vi "SD Card_Read LED  File.vi"() -> ()   [LabVIEW 2015]
doc: "TheSD Card - Read Data - Arduino Target example demonstrates how to read data previously saved in a SD Card Shield and send the data up to a Host VI via serial communication. This VI will run embedded in the Arduino target.\nTo save data in the SD Card Shield, refer to the SD Card - Log Data.vi shipping example.\n\n<b>Chip Select Pin</b>: Refer to your specific SD Card Shield documentation for its Chip Select (CS) pin number."
uses:
  <vilib>/Aledyne-TSXperts/Arduino Compatible Compiler for LabVIEW/Code Generator/Arduino APIs/Serial/Serial Settings.ctl
  <vilib>/Aledyne-TSXperts/Arduino Compatible Compiler for LabVIEW/Code Generator/Arduino APIs/SD Card/File Mode.ctl
  <vilib>/Aledyne-TSXperts/Arduino Compatible Compiler for LabVIEW/Arduino Compatible Compiler for LabVIEW.lvlib
panel:
  in  "Chip Select Pin":u8=4
  # "Overview: Demonstrates how to read data previously saved in a SD Card Shield and send the data up to a Host VI via serial communication. This VI will run embedded in the Arduino target.\n\nInstructions:\n1. Make sure the shipping example SD Card - Log Data.vi has been executed first by following its instructions. \n2. Connect the Arduino target to the PC via USB cable\n3. Enter the appropriate Chip Select as indicated in your SD Card Shield\ndocumentation\n4. Open the SD Card - Read Data - Host PC.vi and follow its instuctions\n5. Important:  This VI will be compiled and downloaded via a API call in the SD Card - Read Data - Host PC.vi. There is no need to run this VI through depressing its run button"
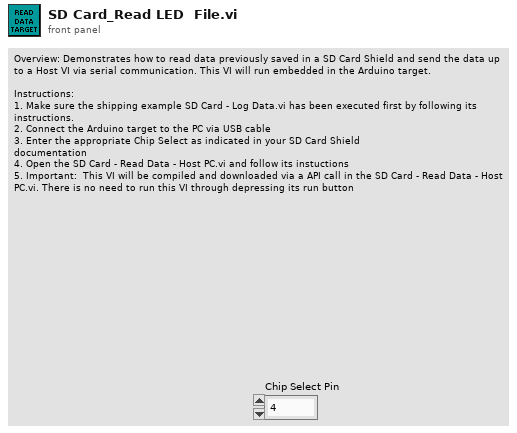
[diagram p1: front panel]
types:
  T1 = typedef "Arduino Compatible Compiler for LabVIEW.lvlib/File Mode.ctl" = enum16{"Read", "Write_Read"}
  T2 = typedef "Arduino Compatible Compiler for LabVIEW.lvlib/Serial Settings.ctl" = u16
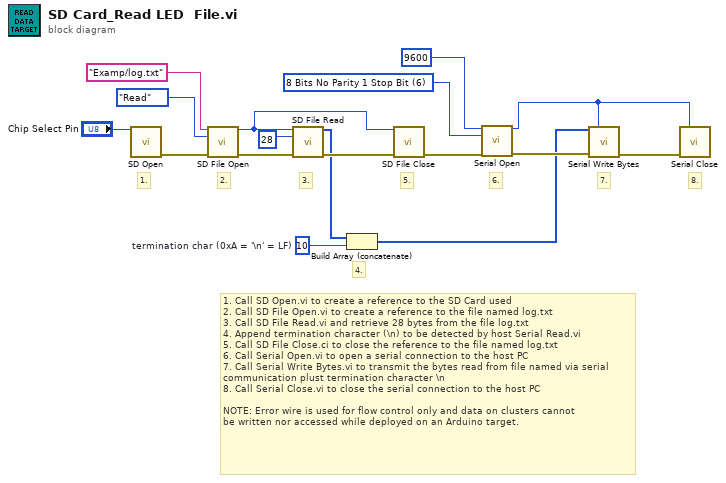
[diagram p0: block diagram]
diagram:
  w1 = u8 10  # termination char (0xA = '\n' = LF)
  w16 = T2 6 items=["5 Bits No Parity 1 Stop Bit"=0, "6 Bits No Parity 1 Stop Bit"=2, "7 Bits No Parity 1 Stop Bit"=4, "8 Bits No Parity 1 Stop Bit"=6, "5 Bits No Parity 2 Stop Bits"=8, "6 Bits No Parity 2 Stop Bits"=10, "7 Bits No Parity 2 Stop Bits"=12, "8 Bits No Parity 2 Stop Bits"=14, "5 Bits Even Parity 1 Stop Bits"=32, "6 Bits Even Parity 1 Stop Bits"=34, "7 Bits Even Parity 1 Stop Bits"=36, "8 Bits Even Parity 1 Stop Bits"=38, "5 Bits Even Parity 2 Stop Bits"=40, "6 Bits Even Parity 2 Stop Bits"=42, "7 Bits Even Parity 2 Stop Bits"=44, "8 Bits Even Parity 2 Stop Bits"=46, "5 Bits Odd Parity 1 Stop Bits"=48, "6 Bits Odd Parity 1 Stop Bits"=50, "7 Bits Odd Parity 1 Stop Bits"=52, "8 Bits Odd Parity 1 Stop Bits"=54, "5 Bits Odd Parity 2 Stop Bits"=56, "6 Bits Odd Parity 2 Stop Bits"=58, "7 Bits Odd Parity 2 Stop Bits"=60, "8 Bits Odd Parity 2 Stop Bits"=62] ("Serial Settings")
  # "7."
  # "6."
  # "5."
  # "4."
  # "8."
  # "3."
  # "2."
  # "1."
  # "1. Call SD Open.vi to create a reference to the SD Card used\n2. Call SD File Open.vi to create a reference to the file named log.txt\n3. Call SD File Read.vi and retrieve 28 bytes from the file log.txt\n4. Append termination character (\\n) to be detected by host Serial Read.vi\n5. Call SD File Close.ci to close the reference to the file named log.txt\n6. Call Serial Open.vi to open a serial connection to the host PC\n7. Call Serial Write Bytes.vi to transmit the bytes read from file named via serial\ncommunication plust termination character \\n\n8. Call Serial Close.vi to close the serial connection to the host PC\n\nNOTE: Error wire is used for flow control only and data on clusters cannot\nbe written nor accessed while deployed on an Arduino target."
  n1 = call <vilib>:"SD Open.vi"("CS Pin"="Chip Select Pin") -> ("error out"=w4:errorcluster)  [unwired: 13 in, 1 out]
  n2 = call <vilib>:"SD File Open.vi"("File"="Examp/log.txt" ("Directory"), "Mode"=File_Mode."Read", "error in (no error)"=w4) -> ("File Reference"=w12:i32, "error out"=w14:errorcluster)  [unwired: 10 in, 1 out]
  n3 = call <vilib>:"SD File Read.vi"("Reference"=w12, "Length"=28, "error in (no error)"=w14) -> ("Data"=w8:u8[], "error out"=w13:errorcluster)  [unwired: 11 in]
  n4 = Build Array (concatenate)(w8, w1) -> (w2:u8[])
  n5 = call <vilib>:"SD File Close.vi"("Reference"=w12, "error in (no error)"=w13) -> ("error out"=w10:errorcluster)  [unwired: 13 in]
  n6 = call <vilib>:"Serial Open.vi"("Speed"=u32 9600, "Serial Settings"=w16, "error in (no error)"=w10) -> ("Instance"=w6:u8, "error out"=w3:errorcluster)  [unwired: 11 in]
  n7 = call <vilib>:"Serial Write Bytes.vi"("Data"=w2, "Instance"=w6, "error in (no error)"=w3) -> ("error out"=w7:errorcluster)  [unwired: 12 in]
  n8 = call <vilib>:"Serial Close.vi"("Instance"=w6, "error in (no error)"=w7) -> ()  [unwired: 13 in, 1 out]
